vi "Galvo Module.vi"(5 "sample mode":i32(ring)=10178 items=["Finite Samples"=10178, "Continuous Samples"=10123, "Hardware Timed Single Point"=12522], 7 "Action":T1(ring)=enum."Init: Calc scan pattern", 8 "error in (no error)":errorcluster, 10 "System Parameters":T2={"Optical Parameters"={"Obj. Focal Length [mm]"=45.0, "Scan Lens EFL[mm]"=60.0, "Tube Lens EFL[mm]"=180.0, "Galvo V Range (+/-)"=10.0, "Galvo Max Half Angle [Deg]"=19.0, "Max Galvo Range[%]"=0.0}, "Vibratome"={"Z Bottom [mm]"=0.0, "Pre Cut Dwell [s]"=0.0, "Blade Frequency [RPM]"=0, "Slice Speed [mm/s]"=0.0, "Post Cut Dwell [s]"=0.0, "Ramp Time [s]"=0.0, "Start X [mm]"=0.0, "Start Y [mm]"=0.0, "Slice Length [mm]"=0.0, "Slice Axis"=enum."Y Axis", "Controller VISA Ref"="COM4"}, "Table Stages"={"X Stage"={"Position"=0.0, "Is.Enabled?"=FALSE, "Is.Connected?"=FALSE, "Device SN"="45876539", "AccelerationMaximum"=0.0, "VelocityMaximum"=0.0, "Acceleration"=0.0, "Velocity"=0.0, "waitTimeout (ms)"=0, "Model"=enum."None", "Is.Homed?"=FALSE}, "Y Stage"={"Position"=0.0, "Is.Enabled?"=FALSE, "Is.Connected?"=FALSE, "Device SN"="45876539", "AccelerationMaximum"=0.0, "VelocityMaximum"=0.0, "Acceleration"=0.0, "Velocity"=0.0, "waitTimeout (ms)"=0, "Model"=enum."None", "Is.Homed?"=FALSE}, "Z Stage"={"Position"=0.0, "Is.Enabled?"=FALSE, "Is.Connected?"=FALSE, "Device SN"="45876539", "AccelerationMaximum"=0.0, "VelocityMaximum"=0.0, "Acceleration"=0.0, "Velocity"=0.0, "waitTimeout (ms)"=0, "Model"=enum."None", "Is.Homed?"=FALSE}}, "Imaging Parameter"={"Raster Scan Direction"=enum."Uni Directional", "Pixel Dwell Time [Clock Cycles]"=1, "Flyback Time [Clock Cycles]"=10, "XY Center [um]"={"X"=1.0, "Y"=1.0}, "Pixel Step Size [um]"=50.0, "XY Image Size"=enum."256 x 256", "Custom"=TRUE, "Custom Size"={"X"=10, "Y"=10}, "Line Averages"=1}, "Galvo HW Parameters"={"Analog Out Channel"="GalvoCtrl/ao0,GalvoCtrl/ao1", "Min Voltage"=-10.0, "Max Voltage"=10.0, "Pixel Clock Source"="/GalvoCtrl/PFI0", "Sample Rate"=1000.0, "Line Clock Out Ch"="GalvoCtrl/port0/line0"}, "Alazar parameters"={"Trigger Settings"={"General Trigger Settings"={"Trigger Operation"=0, "Coupling ID"=2, "Range ID"=2, "Delay"=0, "Timeout Ticks"=0, "Mode"=1, "Parameter"=1}, "Trigger Engine 1"={"Trigger Engine"=0, "Source"=2, "Slope"=1, "Level"=140}, "Trigger Engine 2"={"Trigger Engine"=1000, "Source"=4294967295, "Slope"=1, "Level"=2048}}, "Capture Clock"={"Sample Rate"=100, "Decimation"=0, "Source"=2, "Edge"=0}, "Device ID"={"System ID"=1, "Board ID"=1}, "Ch A Input Control"={"Channel"=1, "Coupling"=2, "Range"=10, "Impedance"=2}, "Ch B Input Control"={"Channel"=2, "Coupling"=2, "Range"=10, "Impedance"=2}, "Acq Settings"={"Window Type"=1, "Record Length"=1440, "Footer"=0, "Offset"=0, "Records Per Buffer"=2048, "Samples per record"=2048, "Records Count (Records/Acq)"=2147483647, "Output Format"=10}}, "Mosaic Paramter"={"X Axis"={"Start [mm]"=0.0, "Steps [pts]"=0.0, "End [mm]"=0.0}, "Y Axis"={"Start [mm]"=0.0, "Steps [pts]"=0.0, "End [mm]"=0.0}, "Scan Pattern"=enum."Uni-directional", "Overlap Options"={"Overlap Type"=enum."No Overlap", "Percent Overlap"=0, "Justify"=enum."Start"}}, "Vibratome Axis"={"Start [mm]"=95.8, "thick[um]"=2.1, "#slices"=111}} {"Alazar parameters"."Acq Settings"."Output Format" items=["U16_LOG"=1, "U16_AMP2"=257]; "Alazar parameters"."Acq Settings"."Window Type" items=["DSP_WINDOW_NONE", "DSP_WINDOW_HANNING", "DSP_WINDOW_HAMMING", "DSP_WINDOW_BLACKMAN", "DSP_WINDOW_BLACKMAN_HARRIS", "DSP_WINDOW_BARTLETT"]; "Alazar parameters"."Acq Settings"."Footer" items=["FOOTER_NONE", "FOOTER_NPT"]; "Alazar parameters"."Ch B Input Control"."Channel" items=["A"=1, "B"=2, "C"=4, "D"=8]; "Alazar parameters"."Ch B Input Control"."Coupling" items=["AC"=1, "DC"=2]; "Alazar parameters"."Ch B Input Control"."Range" items=["20 mV"=1, "40 mV"=2, "50 mV"=3, "80 mV"=4, "100 mV"=5, "200 mV"=6, "400 mV"=7, "500 mV"=8, "800 mV"=9, "1 V"=10, "1.25 V"=33, "2 V"=11, "4 V"=12, "5 V"=13, "8 V"=14, "10 V"=15, "20 V"=16]; "Alazar parameters"."Ch B Input Control"."Impedance" items=["1 MOhm"=1, "50 Ohm"=2, ""=0]; "Alazar parameters"."Ch A Input Control"."Channel" items=["A"=1, "B"=2, "C"=4, "D"=8]; "Alazar parameters"."Ch A Input Control"."Coupling" items=["AC"=1, "DC"=2]; "Alazar parameters"."Ch A Input Control"."Range" items=["20 mV"=1, "40 mV"=2, "50 mV"=3, "80 mV"=4, "100 mV"=5, "200 mV"=6, "400 mV"=7, "500 mV"=8, "800 mV"=9, "1 V"=10, "1.25 V"=33, "2 V"=11, "4 V"=12, "5 V"=13, "8 V"=14, "10 V"=15, "20 V"=16]; "Alazar parameters"."Ch A Input Control"."Impedance" items=["1 MOhm"=1, "50 Ohm"=2, ""=0]; "Alazar parameters"."Capture Clock"."Edge" items=["Rising", "Falling"]; "Alazar parameters"."Capture Clock"."Source" items=["Internal"=1, "Fast External"=2, "Medium External"=3, "Slow External"=4, "External AC"=5, "External DC"=6, "External 10MHz"=7]; "Alazar parameters"."Trigger Settings"."General Trigger Settings"."Trigger Operation" items=["J", "K", "J OR K", "J AND K", "J XOR K", "J AND NOT K", "NOT J AND K"]; "Alazar parameters"."Trigger Settings"."General Trigger Settings"."Coupling ID" items=["AC"=1, "DC"=2]; "Alazar parameters"."Trigger Settings"."General Trigger Settings"."Range ID" items=["5 V", "1 V", "TTL"]; "Alazar parameters"."Trigger Settings"."Trigger Engine 1"."Trigger Engine" items=["J", "K"]; "Alazar parameters"."Trigger Settings"."Trigger Engine 1"."Source" items=["A", "B", "External", "Disable", "C", "D"]; "Alazar parameters"."Trigger Settings"."Trigger Engine 1"."Slope" items=["Positive"=1, "Negative"=2]; "Alazar parameters"."Trigger Settings"."Trigger Engine 2"."Trigger Engine" items=["J", "K"]; "Alazar parameters"."Trigger Settings"."Trigger Engine 2"."Source" items=["A", "B", "External", "Disable", "C", "D"]; "Alazar parameters"."Trigger Settings"."Trigger Engine 2"."Slope" items=["Positive"=1, "Negative"=2]; "Imaging Parameter"."Line Averages" min=1 max=30 step=1; "Imaging Parameter"."Flyback Time [Clock Cycles]" max=10 step=1; "Imaging Parameter"."Pixel Step Size [um]" min=0.0 max=10.0 step=0.01; "Imaging Parameter"."Custom Size"."Y" min=1 max=30 step=1; "Imaging Parameter"."Custom Size"."X" min=1 max=30 step=1; "Imaging Parameter"."XY Center [um]"."Y" min=1.0 max=30.0 step=1.0; "Imaging Parameter"."XY Center [um]"."X" min=1.0 max=30.0 step=1.0; "Imaging Parameter"."Pixel Dwell Time [Clock Cycles]" max=10 step=1}) -> (0 "error out":errorcluster, 1 "task done?":bool)   [LabVIEW 2018]
uses:
  Controls/System Parameters.ctl
  Controls/Optical Parameters.ctl
  Controls/Vibratome Parameters.ctl
  Controls/Translation Stage Parameters.ctl
  Hardware Mfg/Thorlabs Translation Stages/Controls/Translation Stage Cluster.ctl
  Controls/Translation Stage Types.ctl
  Controls/Imaging Parameters.ctl
  Controls/Scan Direction.ctl
  type defines/Alazar parameters.ctl
  Hardware Mfg/AlazarTech SDK/Controls/General Trigger Settings.ctl
  Hardware Mfg/AlazarTech SDK/Controls/Trigger Engine Controls.ctl
  Hardware Mfg/AlazarTech SDK/Controls/Clock Controls.ctl
  Hardware Mfg/AlazarTech SDK/Controls/Alazar Device ID.ctl
  Hardware Mfg/AlazarTech SDK/Controls/Channel Input Controls.ctl
  Hardware Mfg/AlazarTech SDK/Controls/Alazar Acquisition Settings.ctl
  <vilib>/DAQmx/write.llb/DAQmx Write (Digital 1D U32 1Chan NSamp).vi
  <vilib>/DAQmx/write.llb/DAQmx Write (Analog 2D DBL NChan NSamp).vi
  <vilib>/DAQmx/create/channels.llb/DAQmx Create Channel (DO-Digital Output).vi
  <vilib>/DAQmx/configure/timing.llb/DAQmx Timing (Sample Clock).vi
  <vilib>/DAQmx/create/channels.llb/DAQmx Create Channel (AO-Voltage-Basic).vi
  <vilib>/DAQmx/miscellaneous.llb/DAQmx Fill In Error Info.vi
  <resource>/objmgr/daqmx.rc
panel:
  # "X"
  # "X"
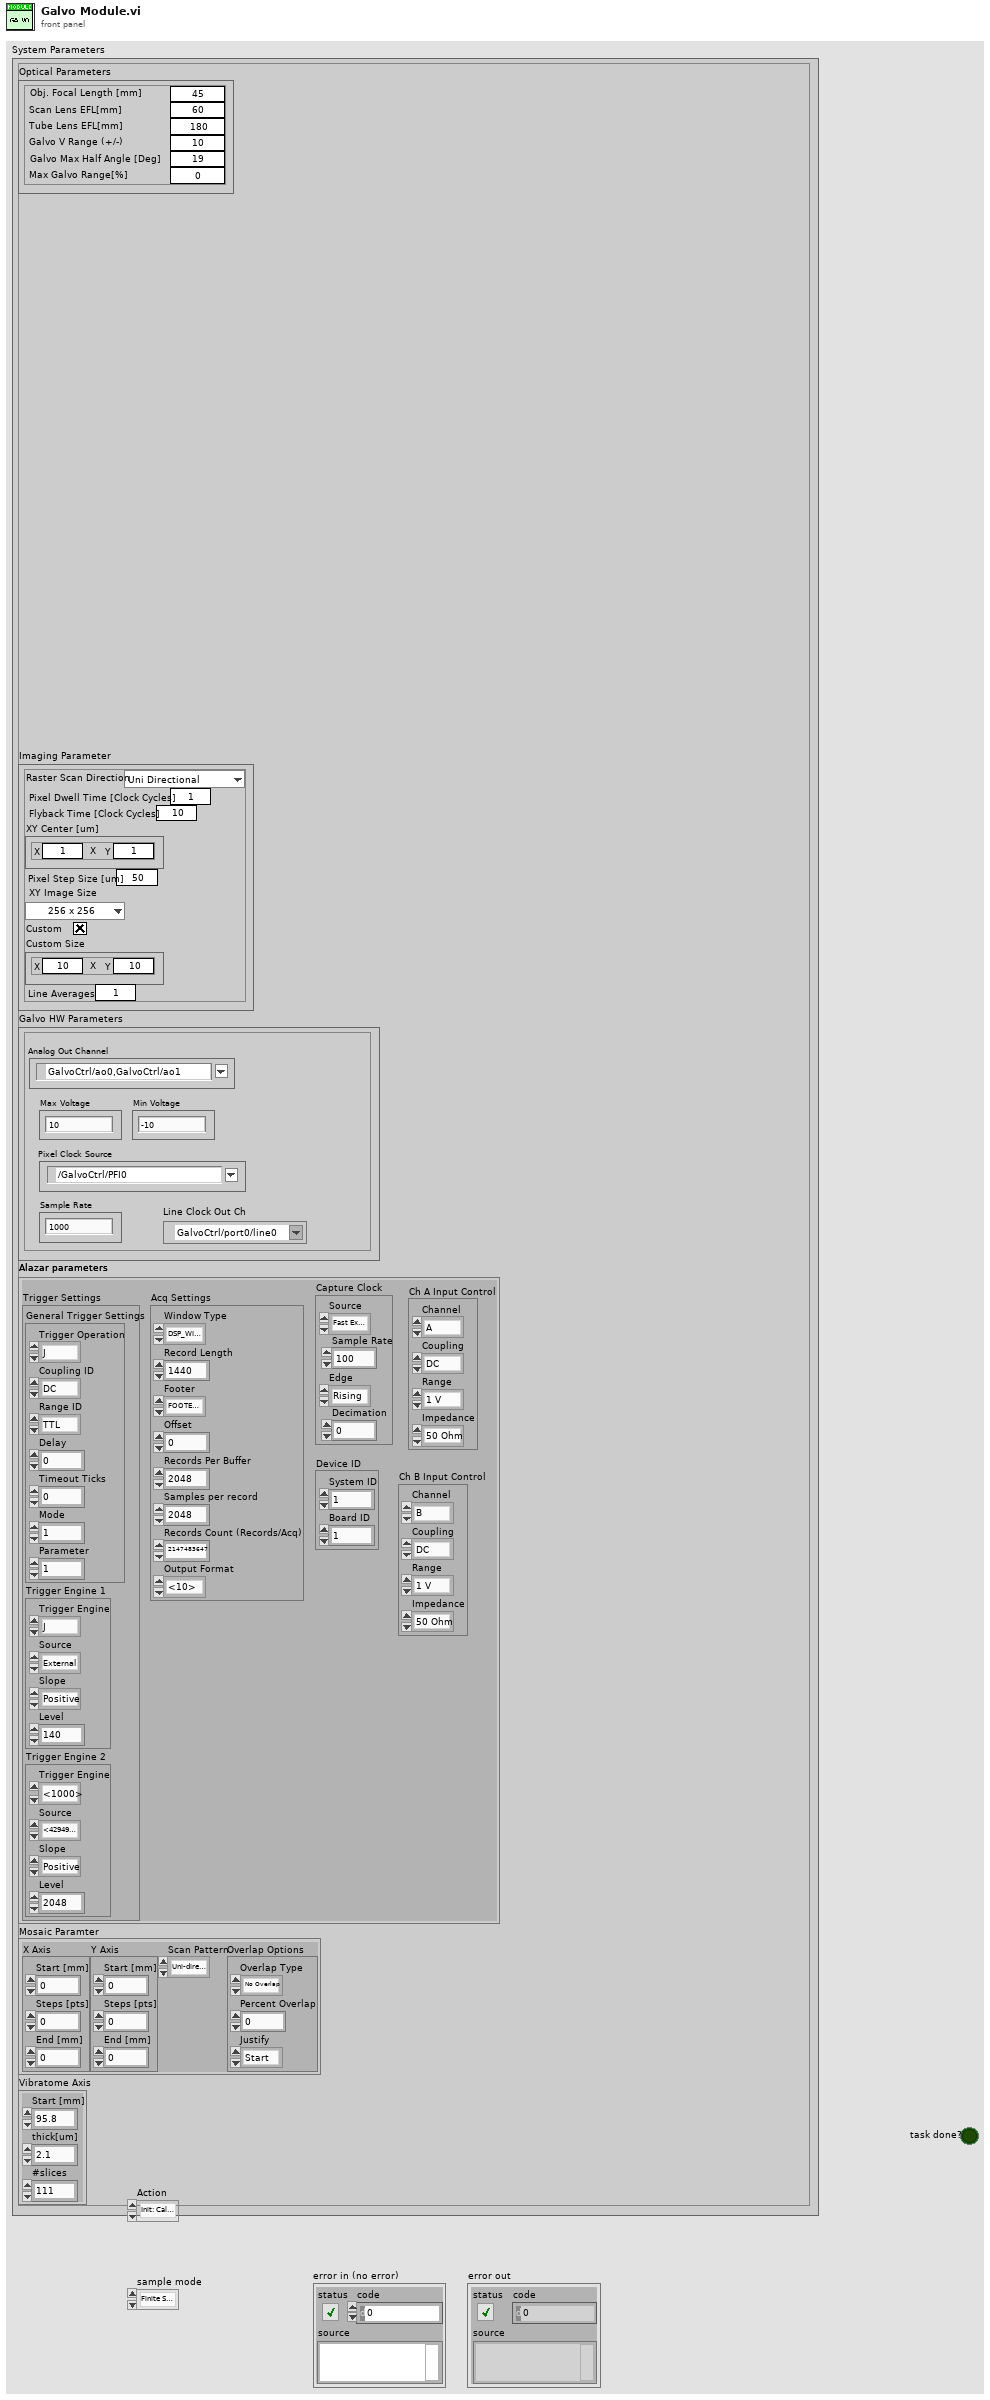
[diagram p1: front panel]
types:
  T1 = enum16{"Configure channels", "Write Scan Pattern", "Start Galvo Task", "Is Task Done?", "Stop Galvo", "Uninit", "Init: Calc scan pattern"}
  T2 = typedef "System Parameters.ctl" = cluster{"Optical Parameters":T3, "Vibratome":T4, "Table Stages":T5, "Imaging Parameter":T8, "Galvo HW Parameters":cluster{"Analog Out Channel":tag, "Min Voltage":dbl, "Max Voltage":dbl, "Pixel Clock Source":tag, "Sample Rate":dbl, "Line Clock Out Ch":tag}, "Alazar parameters":T10, "Mosaic Paramter":cluster{"X Axis":cluster{"Start [mm]":dbl, "Steps [pts]":dbl, "End [mm]":dbl}, "Y Axis":cluster{"Start [mm]":dbl, "Steps [pts]":dbl, "End [mm]":dbl}, "Scan Pattern":enum16{"Uni-directional", "Bi-Directional", "Spiral Out", "Spiral In"}, "Overlap Options":cluster{"Overlap Type":enum16{"No Overlap", "X Only", "Y Only", "X and Y"}, "Percent Overlap":u8, "Justify":enum16{"Start", "Center", "End"}}}, "Vibratome Axis":cluster{"Start [mm]":dbl, "thick[um]":dbl, "#slices":u16}}
  T3 = typedef "Optical Parameters.ctl" = cluster{"Obj. Focal Length [mm]":dbl, "Scan Lens EFL[mm]":dbl, "Tube Lens EFL[mm]":dbl, "Galvo V Range (+/-)":dbl, "Galvo Max Half Angle [Deg]":dbl, "Max Galvo Range[%]":dbl}
  T4 = typedef "Vibratome Parameters.ctl" = cluster{"Z Bottom [mm]":dbl, "Pre Cut Dwell [s]":dbl, "Blade Frequency [RPM]":u16, "Slice Speed [mm/s]":dbl, "Post Cut Dwell [s]":dbl, "Ramp Time [s]":dbl, "Start X [mm]":dbl, "Start Y [mm]":dbl, "Slice Length [mm]":dbl, "Slice Axis":enum16{"X Axis", "Y Axis", "Z Axis"}, "Controller VISA Ref":refnum<visa-resource-name>}
  T5 = typedef "Translation Stage Parameters.ctl" = cluster{"X Stage":T6, "Y Stage":T6, "Z Stage":T6}
  T6 = typedef "Translation Stage Cluster.ctl" = cluster{"Position":dbl, "Is.Enabled?":bool, "Is.Connected?":bool, "Device SN":string, "AccelerationMaximum":dbl, "VelocityMaximum":dbl, "Acceleration":dbl, "Velocity":dbl, "waitTimeout (ms)":i32, "Model":T7, "Is.Homed?":bool}
  T7 = typedef "Translation Stage Types.ctl" = enum16{"None", "Thorlabs LTS", "Thorlabs MLJ"}
  T8 = typedef "Imaging Parameters.ctl" = cluster{"Raster Scan Direction":T9, "Pixel Dwell Time [Clock Cycles]":u16, "Flyback Time [Clock Cycles]":u16, "XY Center [um]":cluster{"X":dbl, "Y":dbl}, "Pixel Step Size [um]":dbl, "XY Image Size":enum16{"32 x 32", "64 x 64", "128 x 128", "256 x 256", "512 x 512", "1024 x 1024", "2048 x 2048"}, "Custom":bool, "Custom Size":cluster{"X":u16, "Y":u16}, "Line Averages":u8}
  T9 = typedef "Scan Direction.ctl" = enum16{"Uni Directional", "Bi Directional", "None"}
  T10 = typedef "Alazar parameters.ctl" = cluster{"Trigger Settings":cluster{"General Trigger Settings":T11, "Trigger Engine 1":T12, "Trigger Engine 2":T12}, "Capture Clock":T13, "Device ID":T14, "Ch A Input Control":T15, "Ch B Input Control":T15, "Acq Settings":T16}
  T11 = typedef "General Trigger Settings.ctl" = cluster{"Trigger Operation":u32, "Coupling ID":u32, "Range ID":u32, "Delay":u32, "Timeout Ticks":u32, "Mode":u32, "Parameter":u32}
  T12 = typedef "Trigger Engine Controls.ctl" = cluster{"Trigger Engine":u32, "Source":u32, "Slope":u32, "Level":u32}
  T13 = typedef "Clock Controls.ctl" = cluster{"Sample Rate":u32, "Decimation":u32, "Source":u32, "Edge":u32}
  T14 = typedef "Alazar Device ID.ctl" = cluster{"System ID":u32, "Board ID":u32}
  T15 = typedef "Channel Input Controls.ctl" = cluster{"Channel":u8, "Coupling":u32, "Range":u32, "Impedance":u32}
  T16 = typedef "Alazar Acquisition Settings.ctl" = cluster{"Window Type":u32, "Record Length":u32, "Footer":u32, "Offset":u32, "Records Per Buffer":u32, "Samples per record":u32, "Records Count (Records/Acq)":u32, "Output Format":u32}
  T17 = cluster{"Analog Out Channel":tag, "Min Voltage":dbl, "Max Voltage":dbl, "Pixel Clock Source":tag, "Sample Rate":dbl, "Line Clock Out Ch":tag}
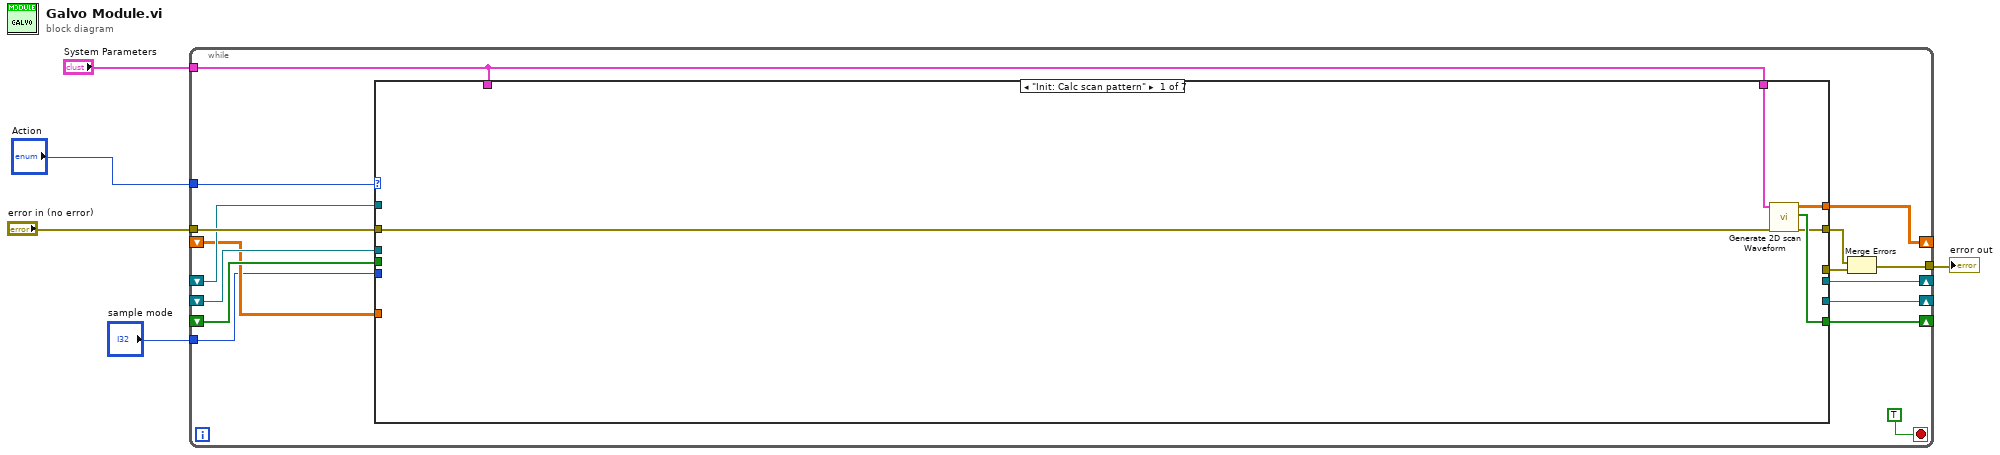
[diagram p0: block diagram]
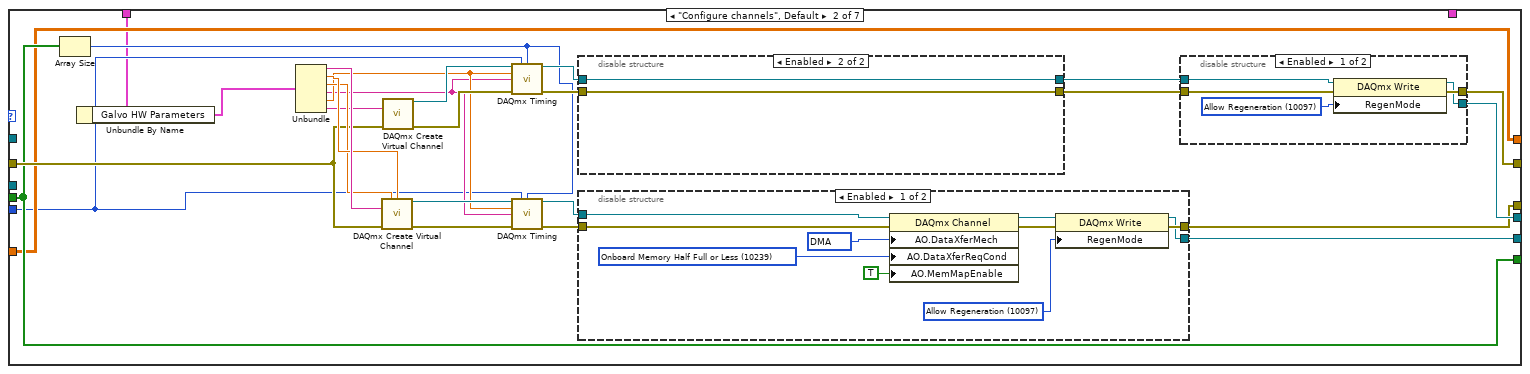
[diagram p2: hidden frame]
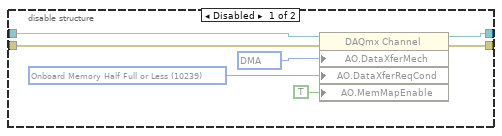
[diagram p5: hidden frame]
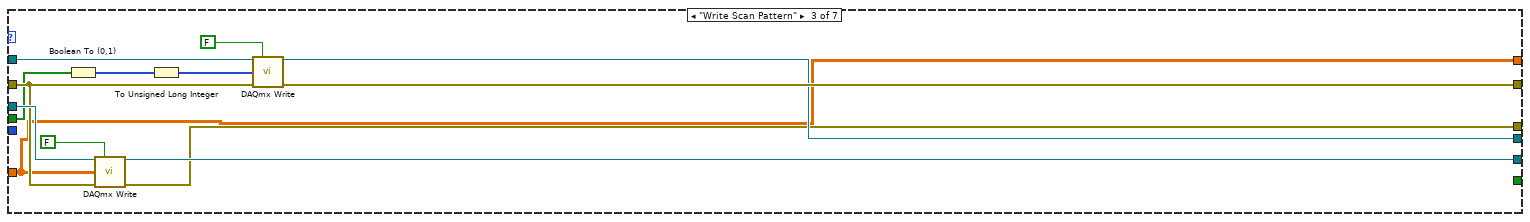
[diagram p6: hidden frame]
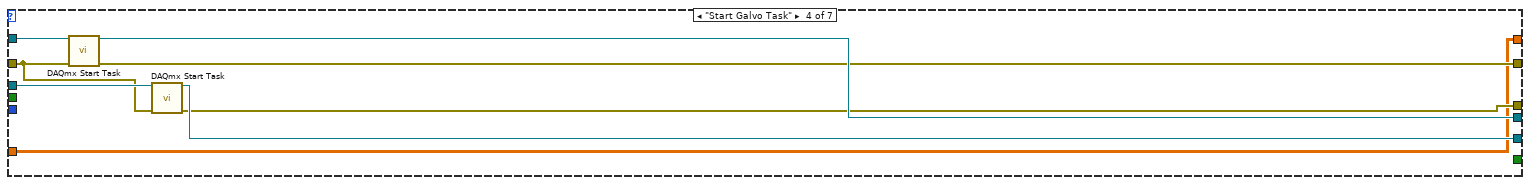
[diagram p7: hidden frame]
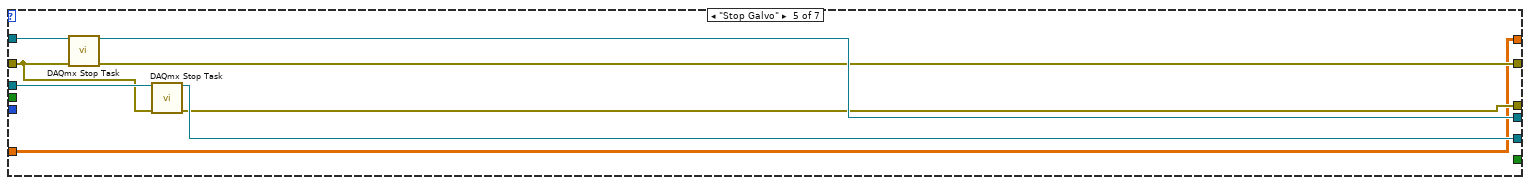
[diagram p8: hidden frame]
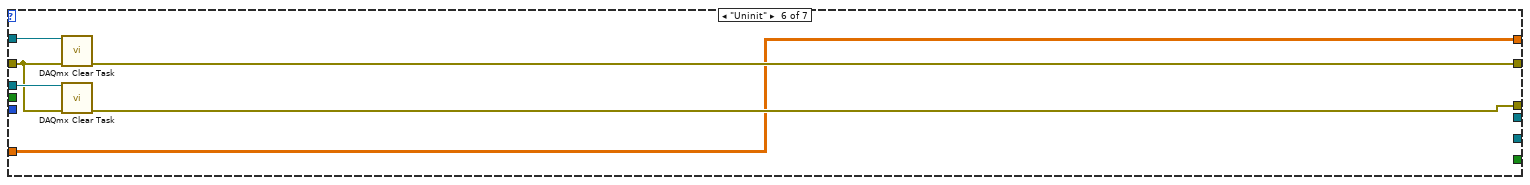
[diagram p9: hidden frame]
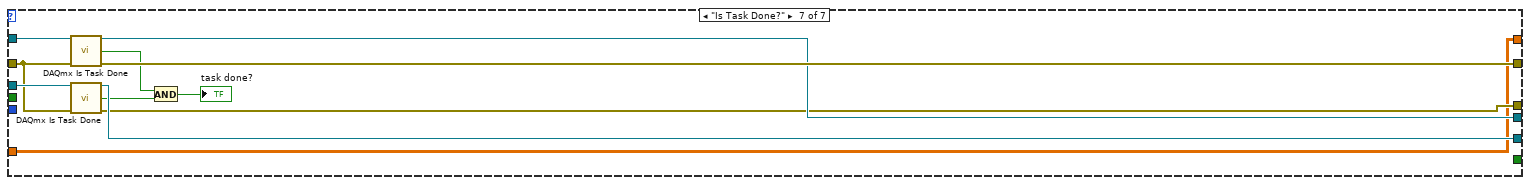
[diagram p10: hidden frame]
diagram:
  n1 = while {
    tunnel: "Action" -> [w21]
    shift-right: [w20] -> _
    shift-left: _ -> [w19]
    tunnel: [w16] -> w4
    tunnel: "error in (no error)" -> [w18]
    shift-right: [w14] -> _
    shift-left: _ -> [w13]
    shift-right: [w12] -> _
    shift-left: _ -> [w9]
    shift-right: [w11] -> _
    shift-left: _ -> [w10]
    tunnel: "sample mode" -> [w8]
    tunnel: "System Parameters" -> [w6]
    stop <- TRUE stop-if-true
    n2 = case shown="\"Init: Calc scan pattern\"" w21 {
      tunnel: [_ w48 w86 w101 w109 _ w126] -> w20
      tunnel: w19 -> [_ _ w94 w102 w110 w116 w127]
      tunnel: w18 -> [w23 w44 w91 w100 w108 w113 w123]
      tunnel: [w24 w36 w90 w97 w105 w115 w122] -> w15
      tunnel: [_ w35 w88 w98 w106 _ w119] -> w14
      tunnel: w13 -> [_ _ w87 w99 w107 w114 w124]
      tunnel: [w26 w32 w82 w95 w103 w111 w117] -> w12
      tunnel: [w25 w33 _ _ _ _ _] -> w11
      tunnel: w10 -> [_ w33 w85 _ _ _ _]
      tunnel: w9 -> [_ w32 w82 w95 w103 w111 w117]
      tunnel: w8 -> [_ w30 _ _ _ _ _]
      tunnel: [_ w29 w83 w96 w104 w112 w118] -> w7
      tunnel: w6 -> [w22 _ _ _ _ _ _]
      tunnel: w6 -> [_ w28 _ _ _ _ _]
      frame "Init: Calc scan pattern" {
        n3 = call "Generate 2D scan Waveform.vi"("error in (no error)"=w23, "System Parameters [In]"=w22) -> ("error out"=w24:errorcluster, "Digital Line Acq"=w25:bool[], "XY"=w26:dbl[][])  [unwired: 4 in, 3 out]
      }
      frame "Configure channels", Default {
        n4 = Array Size(array=w33) -> (size(s)=w31:i32)
        n5 = Unbundle By Name(w28) -> ("Galvo HW Parameters"=w27:T17)
        n6 = Unbundle(w27) -> ("Analog Out Channel"=w52:tag, "Min Voltage"=w51:dbl, "Max Voltage"=w50:dbl, "Pixel Clock Source"=w34:tag, "Sample Rate"=w41:dbl, "Line Clock Out Ch"=w47:tag)
        n7 = call-poly <vilib>:"DAQmx Create Virtual Channel.vi"("maximum value"=w50, "minimum value"=w51, "physical channels"=w52, "error in"=w44) -> ("task out"=w46:refnum<k21>, "error out"=w45:errorcluster)  [unwired: 10 in]
        n8 = call-poly <vilib>:"DAQmx Create Virtual Channel.vi"("lines"=w47, "error in"=w44) -> ("task out"=w42:refnum<k21>, "error out"=w43:errorcluster)  [unwired: 12 in]
        n9 = call-poly <vilib>:"DAQmx Timing.vi"("task/channels in"=w42, "sample mode"=w30, "samples per channel"=w31, "rate"=w41, "source"=w34, "error in"=w43) -> ("task out"=w37:refnum<k21>, "error out"=w38:errorcluster)  [unwired: 8 in]
        n10 = call-poly <vilib>:"DAQmx Timing.vi"("task/channels in"=w46, "sample mode"=w30, "samples per channel"=w31, "rate"=w41, "source"=w34, "error in"=w45) -> ("task out"=w49:refnum<k21>, "error out"=w53:errorcluster)  [unwired: 8 in]
        n11 = disable-structure shown="Enabled" {
          disable-tunnel: [w79 w80] -> w40
          disable-tunnel: [w78 w81] -> w39
          disable-tunnel: w38 -> [w74 w81]
          disable-tunnel: w37 -> [w73 w80]
          frame Disabled {
            w76 = 10239 items=["Onboard Memory Empty"=10235, "Onboard Memory Half Full or Less"=10239, "Onboard Memory Less than Full"=10242] ("AO.DataXferReqCond")
            w77 = 10054 items=["DMA"=10054, "Interrupts"=10204, "Programmed I/O"=10264, "USB Bulk"=12590] ("AO.DataXferMech")
            n12 = property class="DAQmx Channel"(reference=w73, error in=w74, "AO.DataXferMech"=w77, "AO.DataXferReqCond"=w76, "AO.MemMapEnable"=TRUE) -> (reference out=w79:refnum<k21>, error out=w78:errorcluster)
          }
          frame Enabled {
          }
        }
        n13 = disable-structure shown="Enabled" {
          disable-tunnel: w53 -> [w70 w71]
          disable-tunnel: w49 -> [w68 w72]
          disable-tunnel: [w64 w71] -> w29
          disable-tunnel: [w61 w72] -> w48
          frame Enabled {
            w62 = 10097 items=["Allow Regeneration"=10097, "Do Not Allow Regeneration"=10158] ("RegenMode")
            w66 = 10239 items=["Onboard Memory Empty"=10235, "Onboard Memory Half Full or Less"=10239, "Onboard Memory Less than Full"=10242] ("AO.DataXferReqCond")
            w67 = 10054 items=["DMA"=10054, "Interrupts"=10204, "Programmed I/O"=10264, "USB Bulk"=12590] ("AO.DataXferMech")
            n14 = property class="DAQmx Channel"(reference=w68, error in=w70, "AO.DataXferMech"=w67, "AO.DataXferReqCond"=w66, "AO.MemMapEnable"=TRUE) -> (reference out=w63:refnum<k21>, error out=w69:errorcluster)
            n15 = property class="DAQmx Write"(reference=w63, error in=w69, "RegenMode"=w62) -> (reference out=w61:refnum<k21>, error out=w64:errorcluster)
          }
          frame Disabled {
          }
        }
        n16 = disable-structure shown="Enabled" {
          disable-tunnel: w40 -> [w58 w60]
          disable-tunnel: w39 -> [w57 w59]
          disable-tunnel: [w55 w59] -> w36
          disable-tunnel: [w54 w60] -> w35
          frame Enabled {
            w56 = 10097 items=["Allow Regeneration"=10097, "Do Not Allow Regeneration"=10158] ("RegenMode")
            n17 = property class="DAQmx Write"(reference=w58, error in=w57, "RegenMode"=w56) -> (reference out=w54:refnum<k21>, error out=w55:errorcluster)
          }
          frame Disabled {
          }
        }
      }
      frame "Write Scan Pattern" {
        n18 = Boolean To (0,1)(Boolean=w85) -> (0, 1=w92:i16[])
        n19 = call-poly <vilib>:"DAQmx Write.vi"("task/channels in"=w94, "auto start"=FALSE, "data"=w82, "error in"=w91) -> ("task out"=w86:refnum<k21>, "error out"=w83:errorcluster)  [unwired: 9 in, 1 out]
        n20 = To Unsigned Long Integer(number=w92) -> (unsigned 32bit integer=w84:u32[])
        n21 = call-poly <vilib>:"DAQmx Write.vi"("task/channels in"=w87, "auto start"=FALSE, "data"=w84, "error in"=w91) -> ("task out"=w88:refnum<k21>, "error out"=w90:errorcluster)  [unwired: 9 in, 1 out]
      }
      frame "Start Galvo Task" {
        n22 = call <vilib>:"DAQmx Start Task.vi"("task/channels in"=w99, "error in"=w100) -> ("task out"=w98:refnum<k21>, "error out"=w97:errorcluster)  [unwired: 12 in]
        n23 = call <vilib>:"DAQmx Start Task.vi"("task/channels in"=w102, "error in"=w100) -> ("task out"=w101:refnum<k21>, "error out"=w96:errorcluster)  [unwired: 12 in]
      }
      frame "Stop Galvo" {
        n24 = call <vilib>:"DAQmx Stop Task.vi"("task/channels in"=w107, "error in"=w108) -> ("task out"=w106:refnum<k21>, "error out"=w105:errorcluster)  [unwired: 12 in]
        n25 = call <vilib>:"DAQmx Stop Task.vi"("task/channels in"=w110, "error in"=w108) -> ("task out"=w109:refnum<k21>, "error out"=w104:errorcluster)  [unwired: 12 in]
      }
      frame "Uninit" {
        n26 = call <vilib>:"DAQmx Clear Task.vi"("task in"=w114, "error in"=w113) -> ("error out"=w115:errorcluster)  [unwired: 13 in]
        n27 = call <vilib>:"DAQmx Clear Task.vi"("task in"=w116, "error in"=w113) -> ("error out"=w112:errorcluster)  [unwired: 13 in]
      }
      frame "Is Task Done?" {
        n28 = call <vilib>:"DAQmx Is Task Done.vi"("task/channels in"=w124, "error in"=w123) -> ("task out"=w119:refnum<k21>, "task done?"=w120:bool, "error out"=w122:errorcluster)  [unwired: 11 in]
        n29 = call <vilib>:"DAQmx Is Task Done.vi"("task/channels in"=w127, "error in"=w123) -> ("task out"=w126:refnum<k21>, "task done?"=w125:bool, "error out"=w118:errorcluster)  [unwired: 11 in]
        n30 = And(x=w120, y=w125) -> (x .and. y?=→"task done?":bool)
      }
    }
    n31 = Merge Errors(w15, w7) -> (w16:errorcluster)
  }
  "error out" <- w4
